vi "test 2.vi"() -> ()   [LabVIEW 2009]
panel:
  out "Array":dbl[][](array[numeric])
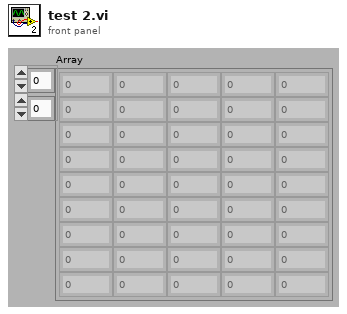
[diagram p1: front panel]
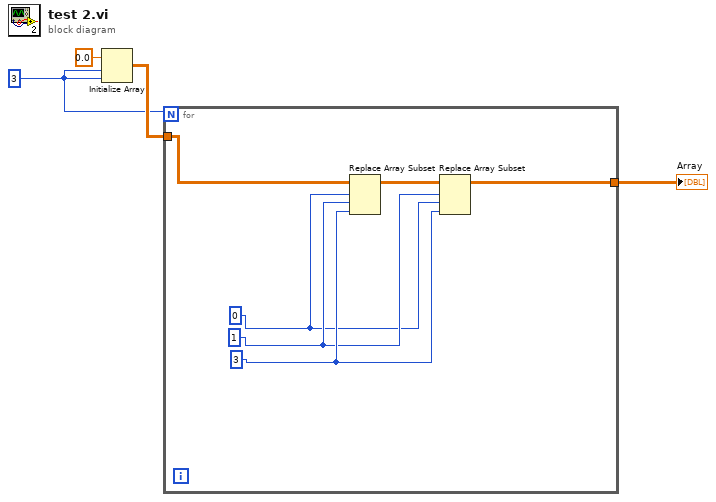
[diagram p0: block diagram]
diagram:
  w1 = 3
  n1 = Initialize Array(0.0 ("element"), w1, w1) -> (w3:dbl[][])
  n2 = for {
    N: w1 -> [_]
    tunnel: w3 -> [w10]
    tunnel: [w8] -> w2
    w7 = 3
    w6 = 1
    w5 = 0
    n3 = Replace Array Subset(array=w10, new element=w7, index (row)=w5, index (col)=w6) -> (w9:dbl[][])
    n4 = Replace Array Subset(array=w9, new element=w7, index (row)=w6, index (col)=w5) -> (w8:dbl[][])
  }
  "Array" <- w2
